vi "getPoints.vi"(0 "reference":refnum<class "ClassRelationshipEdge.lvclass">, 5 "error in (no error)":errorcluster) -> (14 "reference out":refnum<class "ClassRelationshipEdge.lvclass">, 15 "points":T1[](array[typedef]) {"y" format="%.2f"; "x" format="%.2f"}, 19 "error out":errorcluster)   [LabVIEW 2016, in "ClassRelationshipEdge.lvclass"]
uses:
  <resource>/Framework/Providers/Open_GDS/UML/ClassRelationshipEdge_class/ClassRelationshipEdge.lvclass
  C:/Program Files (x86)/National Instruments/LabVIEW 2016/resource/Framework/Providers/Open_GDS/UML/AbstractEdge_class/AbstractEdge.lvclass
  <resource>/Framework/Providers/Open_GDS/UML/General/Point/Point Point2D.ctl
  <resource>/Framework/Providers/Open_GDS/UML/BentStyle_class/BentStyle.lvclass
  <resource>/Framework/Providers/Open_GDS/UML/AbstractNode_class/AbstractNode.lvclass
  <resource>/Framework/Providers/Open_GDS/UML/AbstractEdge_class/AbstractEdge.lvclass
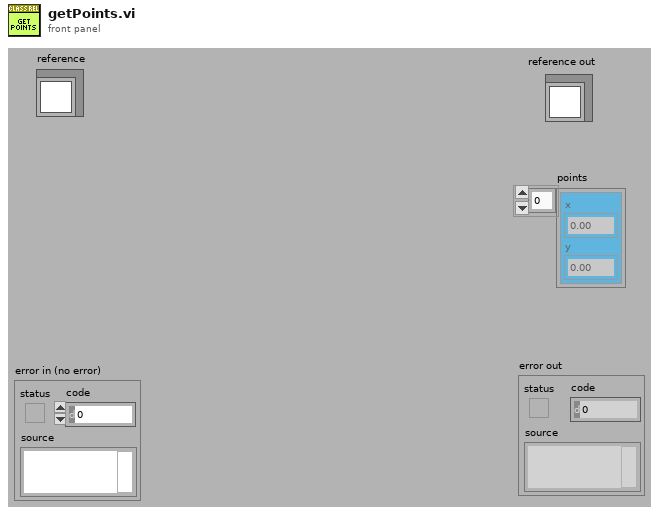
[diagram p1: front panel]
types:
  T1 = typedef "Point Point2D.ctl" = cluster{"x":dbl, "y":dbl}
  T2 = typedef "ClassRelationshipEdge.lvclass/ObjectAttributes.ctl" = cluster{"bentStyleRef":refnum<class "BentStyle.lvclass">, "startConnectionOffset":cluster{"x":i32, "y":i32}, "endConnectionOffset":cluster{"x":i32, "y":i32}, "MidLineOffset":cluster{"x":i32, "y":i32}, "DepClass":T3}
  T3 = typedef "ReversedEngineering_ViDependencyDetailsType.ctl" = cluster{"ThisVIs/Ctls":path[], "Dependent_VIs/Ctls":path[]}
  T4 = typedef "AbstractEdge.lvclass/ObjectAttributes.ctl" = cluster{"start":refnum<class "AbstractNode.lvclass">, "end":refnum<class "AbstractNode.lvclass">}
  T5 = typedef "Rectangle Rectangle2D.ctl" = cluster{"x":dbl, "y":dbl, "width":dbl, "height":dbl}
  T6 = typedef "Direction.lvclass/DirectionTypes.ctl" = enum16{"NORTH", "SOUTH", "EAST", "WEST"}
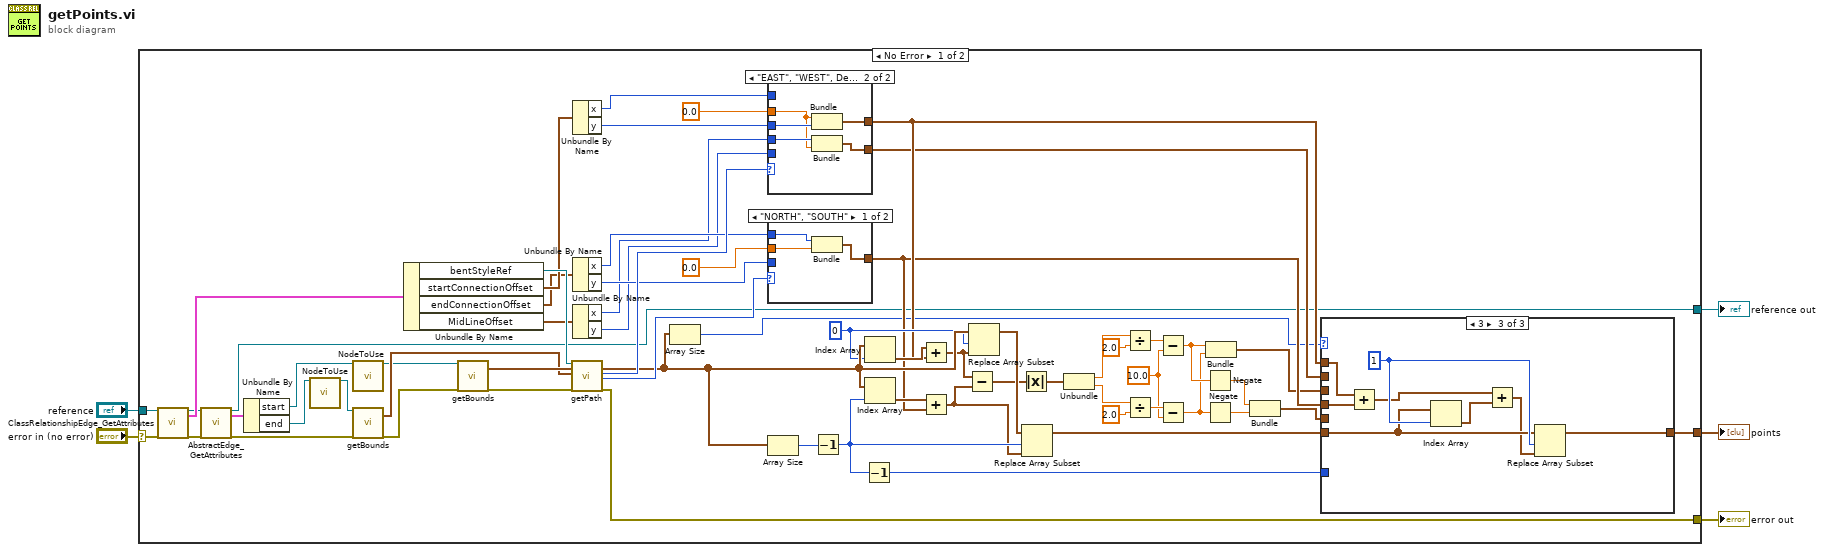
[diagram p0: block diagram]
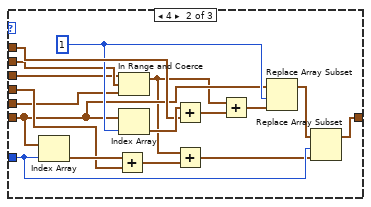
[diagram p3: hidden frame]
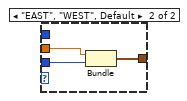
[diagram p4: hidden frame]
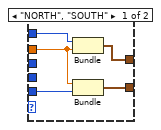
[diagram p5: hidden frame]
diagram:
  n1 = case shown="No Error" "error in (no error)" {
    selector: "error in (no error)" -> [w55 w110]
    tunnel: "reference" -> [w67 w111]
    tunnel: [w56 w110] -> w4
    tunnel: [w7 w111] -> w3
    tunnel: [w57 _] -> w1
    frame No Error {
      w29 = 10.0 ("y")
      w45 = 0 ("index")
      n2 = call <resource>:"ClassRelationshipEdge_GetAttributes.vi"("reference in"=w67, "error in (no error)"=w55) -> ("reference out"=w10:refnum<class "ClassRelationshipEdge.lvclass">, "Data"=w11:T2, "error out"=w9:errorcluster)  [unwired: 1 in, 14 out]
      n3 = call <resource>:"AbstractEdge_GetAttributes.vi"("reference in"=w10, "error in (no error)"=w9) -> ("reference out"=w7:refnum<class "ClassRelationshipEdge.lvclass">, "Data"=w6:T4, "error out"=w8:errorcluster)  [unwired: 14 in, 1 out]
      n4 = Unbundle By Name(w6) -> ("start"=w15:refnum<class "AbstractNode.lvclass">, "end"=w13:refnum<class "AbstractNode.lvclass">)
      n5 = call <resource>:"NodeToUse.vi"("reference in"=w13) -> ("reference out"=w12:refnum<class "AbstractNode.lvclass">)  [unwired: 15 in, 3 out]
      n6 = call <resource>:"NodeToUse.vi"("reference in"=w15) -> ("reference out"=w14:refnum<class "AbstractNode.lvclass">)  [unwired: 15 in, 3 out]
      n7 = call-dynamic "getBounds.vi"("reference"=w12, "error in (no error)"=w8) -> ("bounds"=w63:T5, "error out"=w65:errorcluster)  [unwired: 16 out]
      n8 = Unbundle By Name(w11) -> ("bentStyleRef"=w66:refnum<class "BentStyle.lvclass">, "startConnectionOffset"=w62:cluster{"x":i32, "y":i32}, "endConnectionOffset"=w58:cluster{"x":i32, "y":i32}, "MidLineOffset"=w37:cluster{"x":i32, "y":i32})
      n9 = call-dynamic "getBounds.vi"("reference"=w14, "error in (no error)"=w65) -> ("bounds"=w64:T5, "error out"=w54:errorcluster)  [unwired: 16 out]
      n10 = call-dynamic "getPath.vi"("reference"=w66, "start"=w64, "end"=w63, "error in (no error)"=w54) -> ("path"=w59:T1[], "startDirection"=w61:T6, "endDirection"=w60:T6, "error out"=w56:errorcluster)  [unwired: 12 out]
      n11 = Unbundle By Name(w62) -> ("x"=w50:i32, "y"=w52:i32)
      n12 = Unbundle By Name(w58) -> ("x"=w49:i32, "y"=w47:i32)
      n13 = Unbundle By Name(w37) -> ("x"=w35:i32, "y"=w36:i32)
      n14 = Array Size(array=w59) -> (size(s)=w16:i32)
      n15 = case shown="\"EAST\", \"WEST\", Default" w61 {
        tunnel: w52 -> [_ w109]
        tunnel: 0.0 ("y") -> [w102 w106]
        tunnel: w50 -> [w104 _]
        tunnel: [w103 w108] -> w39
        tunnel: w36 -> [w101 _]
        tunnel: w35 -> [_ w107]
        tunnel: [w100 w105] -> w34
        frame "NORTH", "SOUTH" {
          n16 = Bundle("x"=w104, "y"=w102) -> (w103:cluster{"x":i32, "y":dbl})  [unwired: 1 out]
          n17 = Bundle("y"=w102, "y"=w101) -> (w100:cluster{"y":dbl, "y":i32})  [unwired: 1 out]
        }
        frame "EAST", "WEST", Default {
          n18 = Bundle("y"=w106, "y"=w109) -> (w108:cluster{"y":dbl, "y":i32})  [unwired: 1 out]
          n19 = Bundle("x"=w107, "y"=w106) -> (w105:cluster{"x":i32, "y":dbl})  [unwired: 1 out]
        }
      }
      n20 = case shown="\"NORTH\", \"SOUTH\"" w60 {
        tunnel: w47 -> [_ w99]
        tunnel: 0.0 ("y") -> [w94 w98]
        tunnel: w49 -> [w96 _]
        tunnel: [w95 w97] -> w38
        frame "NORTH", "SOUTH" {
          n21 = Bundle("x"=w96, "y"=w94) -> (w95:cluster{"x":i32, "y":dbl})  [unwired: 1 out]
        }
        frame "EAST", "WEST", Default {
          n22 = Bundle("y"=w98, "y"=w99) -> (w97:cluster{"y":dbl, "y":i32})  [unwired: 1 out]
        }
      }
      n23 = Array Size(array=w59) -> (size(s)=w46:i32)
      n24 = Decrement(x=w46) -> (x-1=w42:i32)
      n25 = Decrement(x=w42) -> (x-1=w40:i32)
      n26 = Index Array(array=w59, index=w45) -> (element=w53:T1)
      n27 = Index Array(array=w59, index=w42) -> (element=w41:T1)
      n28 = Add(x=w53, y=w39) -> (x+y=w21:T1)
      n29 = Add(x=w41, y=w38) -> (x+y=w20:T1)
      n30 = Subtract(x=w21, y=w20) -> (x-y=w22:T1)
      n31 = Replace Array Subset(array=w59, new element=w21, index=w45) -> (w44:T1[])
      n32 = Absolute Value(x=w22) -> (abs(x)=w19:T1)
      n33 = Replace Array Subset(array=w44, new element=w20, index=w42) -> (w43:T1[])
      n34 = Unbundle(w19) -> ("x"=w18:dbl, "y"=w17:dbl)
      n35 = Divide(x=w18, y=2.0) -> (x/y=w32:dbl)
      n36 = Divide(x=w17, y=2.0) -> (x/y=w30:dbl)
      n37 = Subtract(x=w32, y=w29) -> (x-y=w28:dbl)
      n38 = Subtract(x=w30, y=w29) -> (x-y=w27:dbl)
      n39 = Negate(x=w28) -> (-x=w26:dbl)
      n40 = Negate(x=w27) -> (-x=w25:dbl)
      n41 = Bundle(w28, w27) -> (w24:cluster{dbl, dbl})  [unwired: 1 out]
      n42 = Bundle(w26, w25) -> (w23:cluster{dbl, dbl})  [unwired: 1 out]
      n43 = case shown="3" w16 {
        tunnel: w43 -> [w68 w78 w92]
        tunnel: [w68 w84 w91] -> w57
        tunnel: w40 -> [_ w77 _]
        tunnel: w39 -> [_ w82 w90]
        tunnel: w38 -> [_ w79 w89]
        tunnel: w34 -> [_ w72 _]
        tunnel: w24 -> [_ w70 _]
        tunnel: w23 -> [_ w69 _]
        frame 0, Default {
        }
        frame 4 {
          w80 = 1 ("index")
          n44 = Index Array(array=w78, index=w77) -> (element=w81:T1)
          n45 = Add(x=w81, y=w79) -> (x+y=w75:T1)
          n46 = In Range and Coerce(upper limit=w70, x=w72, lower limit=w69) -> (coerced(x)=w71:cluster{"y":dbl, "y":dbl})  [unwired: 1 out]
          n47 = Index Array(array=w78, index=w80) -> (element=w83:T1)
          n48 = Add(x=w83, y=w82) -> (x+y=w76:T1)
          n49 = Add(x=w71, y=w75) -> (x+y=w73:T1)
          n50 = Add(x=w71, y=w76) -> (x+y=w74:T1)
          n51 = Replace Array Subset(array=w78, new element=w74, index=w80) -> (w85:T1[])
          n52 = Replace Array Subset(array=w85, new element=w73, index=w77) -> (w84:T1[])
        }
        frame 3 {
          w93 = 1 ("index")
          n53 = Add(x=w90, y=w89) -> (x+y=w86:cluster{"y":dbl, "y":dbl})
          n54 = Index Array(array=w92, index=w93) -> (element=w88:T1)
          n55 = Add(x=w86, y=w88) -> (x+y=w87:T1)
          n56 = Replace Array Subset(array=w92, new element=w87, index=w93) -> (w91:T1[])
        }
      }
    }
    frame Error {
    }
  }
  "reference out" <- w3
  "error out" <- w4
  "points" <- w1
